vi "Client.vi"(8 "error in":errorcluster, 10 "Measurement Configuration":T2={"function"=0, "range"=1.0, "resolution_digits"=3.5}, 11 "Resource Name":T4={"resource_name"="GPIB0::3::INSTR", "id_query"=FALSE, "reset_device"=TRUE, "simulate"=TRUE}) -> (0 "error out":errorcluster, 2 "Measured Value":T1, 3 "Initialization Status":T3)   [LabVIEW 2020]
uses:
  Instrument Interaction Client/RPC Messages/external_driver_wrapper_InitializeRequest.ctl
  Instrument Interaction Client/RPC Messages/external_driver_wrapper_InitializeResponse.ctl
  Instrument Interaction Client/RPC Messages/external_driver_wrapper_ConfigureMeasurementDigitsRequest.ctl
  Instrument Interaction Client/RPC Messages/external_driver_wrapper_ReadResponse.ctl
  Instrument Interaction Client/RPC Messages/external_driver_wrapper_CloseRequest.ctl
  Instrument Interaction Client/RPC Messages/external_driver_wrapper_ReadRequest.ctl
  Instrument Interaction Client/Instrument Interaction Client.lvlib
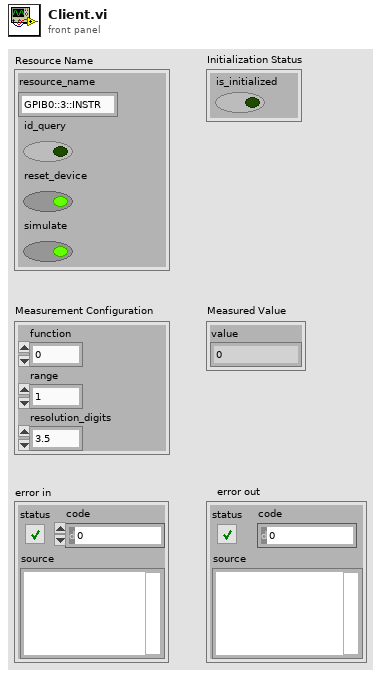
[diagram p1: front panel]
types:
  T1 = typedef "Instrument Interaction Client.lvlib/external_driver_wrapper_ReadResponse.ctl" = cluster{"value":dbl}
  T2 = typedef "Instrument Interaction Client.lvlib/external_driver_wrapper_ConfigureMeasurementDigitsRequest.ctl" = cluster{"function":i32, "range":dbl, "resolution_digits":dbl}
  T3 = typedef "Instrument Interaction Client.lvlib/external_driver_wrapper_InitializeResponse.ctl" = cluster{"is_initialized":bool}
  T4 = typedef "Instrument Interaction Client.lvlib/external_driver_wrapper_InitializeRequest.ctl" = cluster{"resource_name":string, "id_query":bool, "reset_device":bool, "simulate":bool}
  T5 = typedef "Instrument Interaction Client.lvlib/external_driver_wrapper_ReadRequest.ctl" = cluster{"void":string}
  T6 = typedef "Instrument Interaction Client.lvlib/external_driver_wrapper_CloseRequest.ctl" = cluster{"void":string}
  T7 = typedef "grpc-lvsupport-release.lvlib/grpcId.ctl" = u64
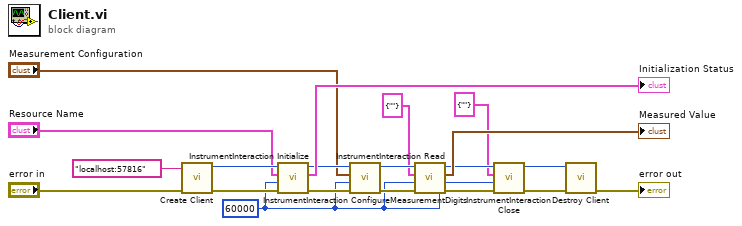
[diagram p0: block diagram]
diagram:
  w2 = 60000 ("timeout (ms)")
  n1 = call "Create Client.vi"("error in"="error in", "address"="localhost:57816") -> ("error out"=w16:errorcluster, "gRPC ID Out"=w18:T7)  [unwired: 8 in]
  n2 = call "InstrumentInteraction Initialize.vi"("error in"=w16, "timeout (ms)"=w2, "Request Data"="Resource Name", "gRPC ID"=w18) -> ("error out"=w12:errorcluster, "Response Data"=→"Initialization Status":T3, "gRPC ID out"=w14:T7)  [unwired: 5 in]
  n3 = call "InstrumentInteraction ConfigureMeasurementDigits.vi"("error in"=w12, "timeout (ms)"=w2, "Request Data"="Measurement Configuration", "gRPC ID"=w14) -> ("error out"=w10:errorcluster, "gRPC ID out"=w11:T7)  [unwired: 5 in, 1 out]
  n4 = call "InstrumentInteraction Read.vi"("error in"=w10, "timeout (ms)"=w2, "Request Data"=T5 {"void"=""}, "gRPC ID"=w11) -> ("error out"=w7:errorcluster, "Response Data"=→"Measured Value":T1, "gRPC ID out"=w8:T7)  [unwired: 5 in]
  n5 = call "InstrumentInteraction Close.vi"("error in"=w7, "timeout (ms)"=w2, "Request Data"=T6 {"void"=""}, "gRPC ID"=w8) -> ("error out"=w5:errorcluster, "gRPC ID out"=w3:T7)  [unwired: 5 in, 1 out]
  n6 = call "Destroy Client.vi"("error in"=w5, "gRPC ID"=w3) -> ("error out"=→"error out":errorcluster)  [unwired: 9 in]
